vi "Write U8 FIFO.vi"(6 "FIFO Timestamps":T1, 8 "error in (no error)":errorcluster, 9 "Timeout (ms)":i32=100, 10 "U8 Data":u8[](array[numeric]), 11 "CIFFIFO in":refnum<class "CIF_NIChn_Fifo_U8.lvclass">) -> (0 "error out":errorcluster, 1 "timed out?":bool, 3 "CIFFIFO out":refnum<class "CIF_NIChn_Fifo_U8.lvclass">)   [LabVIEW 2021, in "CIF_NIChn_Fifo_U8.lvclass"]
uses:
  CIF_NIChn_Fifo_U8.lvclass
  CIF_NIChn_Fifo_U8.lvclass/CIF_NIChn_Fifo_U8.ctl
  CIFChannels/CIFChannels.lvclass
  D:/dev/Packages/Channel_Manager/src/CIFChannels/CIFChannels.lvclass
  ChannelCommon/typedef/TimeStamps.ctl
  ChannelCommon/ChannelCommon.lvlib
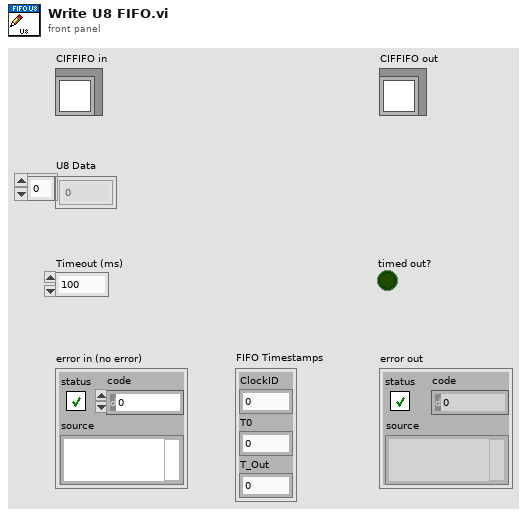
[diagram p1: front panel]
types:
  T1 = typedef "ChannelCommon.lvlib/TimeStamps.ctl" = cluster{"ClockID":u8, "T0":i64, "T_Out":i64}
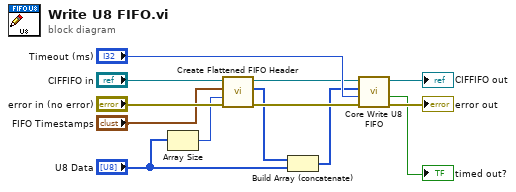
[diagram p0: block diagram]
diagram:
  n1 = Array Size(array="U8 Data") -> (size(s)=w8:i32)
  n2 = call "Create Flattened FIFO Header.vi"("error in (no error)"="error in (no error)", "Data Length"=w8, "FIFO Timestamps"="FIFO Timestamps", "CIFChannels in"="CIFFIFO in") -> ("error out"=w9:errorcluster, "Flattened FIFO Header"=w6:u8[], "CIFChannels out"=w1:refnum<class "CIF_NIChn_Fifo_U8.lvclass">)  [unwired: 5 in]
  n3 = Build Array (concatenate)(w6, "U8 Data") -> (w4:u8[])
  n4 = call "Core Write U8 FIFO.vi"("error in (no error)"=w9, "Timeout (ms)"="Timeout (ms)", "U8 With Header"=w4, "CIFFIFO in"=w1) -> ("error out"=→"error out":errorcluster, "timed out?"=→"timed out?":bool, "CIFFIFO out"=→"CIFFIFO out":refnum<class "CIF_NIChn_Fifo_U8.lvclass">)  [unwired: 5 in]
